vi "Reduce Dielectric Strength Results.vi"(8 "error in (no error)":errorcluster, 11 "Results Array In":string[](array[string])) -> (0 "error out":errorcluster, 1 "Leakage Current":dbl[](array[numeric]), 2 "ACW Current":dbl[](array[numeric]), 3 "ACW Voltage":dbl[](array[numeric]), 4 "Max Leakage Current":dbl, 6 "Min Leakage Current":dbl)   [LabVIEW 2018]
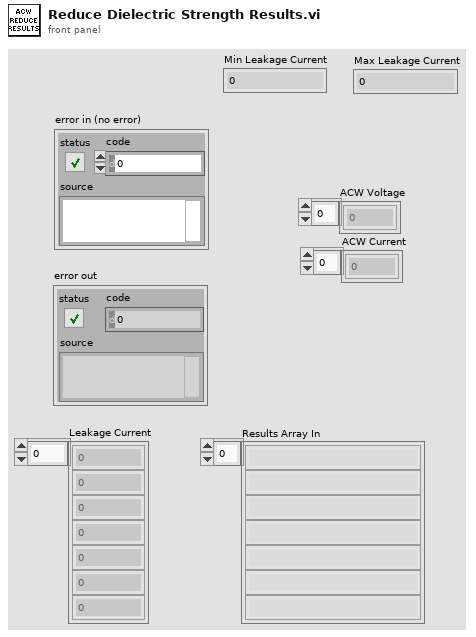
[diagram p1: front panel]
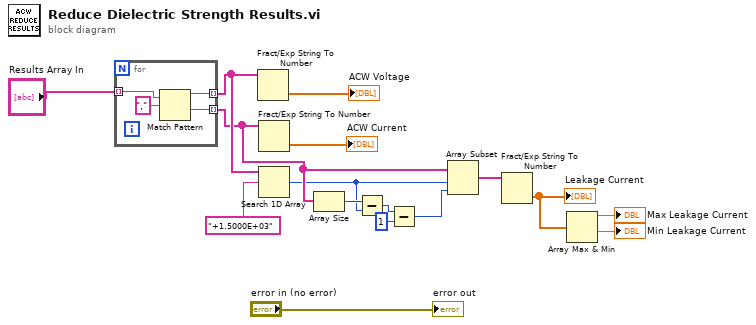
[diagram p0: block diagram]
diagram:
  n1 = for {
    tunnel: "Results Array In" -> [w19] mode=indexing
    tunnel: [w18] -> w15 mode=indexing
    tunnel: [w17] -> w7 mode=indexing
    n2 = Match Pattern(string=w19, regular expression=",") -> (before substring=w18:string, after substring=w17:string)  [unwired: 1 in, 2 out]
  }
  n3 = Fract/Exp String To Number(string=w15) -> (number=→"ACW Voltage":dbl[])  [unwired: 3 in, 1 out]
  n4 = Fract/Exp String To Number(string=w7) -> (number=→"ACW Current":dbl[])  [unwired: 3 in, 1 out]
  n5 = Search 1D Array(1D array=w15, element="+1.5000E+03") -> (index of element=w2:i32)  [unwired: 1 in]
  n6 = Array Size(array=w7) -> (size(s)=w6:i32)
  n7 = Subtract(x=w6, y=w2) -> (x-y=w5:i32)
  n8 = Subtract(x=w5, y=1) -> (x-y=w3:i32)
  n9 = Array Subset(array=w7, index=w2, length=w3) -> (w16:string[])
  n10 = Fract/Exp String To Number(string=w16) -> (number=w12:dbl[])  [unwired: 3 in, 1 out]
  "Leakage Current" <- w12
  n11 = Array Max & Min(array=w12) -> (max value=→"Max Leakage Current":dbl, min value=→"Min Leakage Current":dbl)  [unwired: 2 out]
  "error out" <- "error in (no error)"
